vi "write_params.vi"(8 "error in (no error)":errorcluster caption="entrée d'erreur (pas d'erreur)", 10 "params":T1={"damping"=0.5, "max_iter"=200, "convergence_iter"=15, "copy"=TRUE, "preference"={"preference_type"="None", "preference_list"=[], "preference_float"=0.0}, "affinity"="euclidean", "verbose"=TRUE, "random_state"=0}, 11 "AffinityPropagation en entrée":refnum<class "AffinityPropagation.lvclass">) -> (0 "error out":errorcluster caption="sortie d'erreur", 3 "AffinityPropagation en sortie":refnum<class "AffinityPropagation.lvclass">)   [LabVIEW 2020, in "AffinityPropagation.lvclass"]
uses:
  AffinityPropagation.lvclass
  Controls/affinity_propagation_params.ctl
  AffinityPropagation.lvclass/AffinityPropagation.ctl
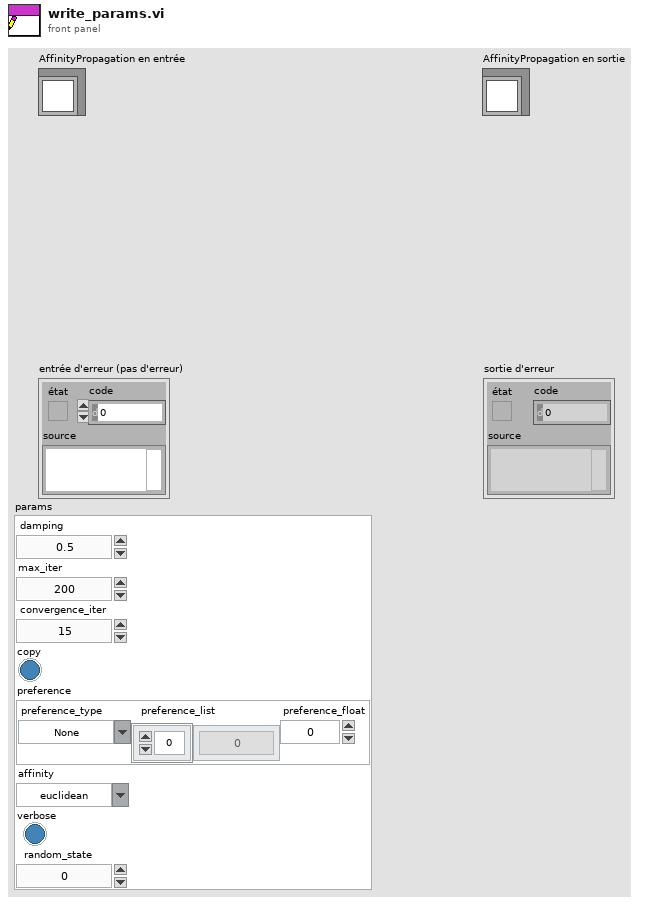
[diagram p1: front panel]
types:
  T1 = typedef "affinity_propagation_params.ctl" = cluster{"damping":dbl, "max_iter":i32, "convergence_iter":i32, "copy":bool, "preference":cluster{"preference_type":string, "preference_list":dbl[], "preference_float":dbl}, "affinity":string, "verbose":bool, "random_state":i32}
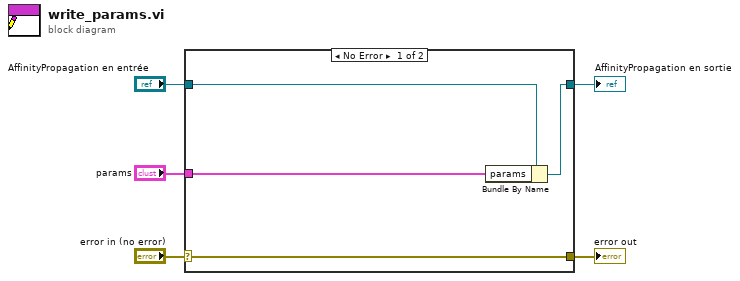
[diagram p0: block diagram]
diagram:
  n1 = case shown="No Error" "error in (no error)" {
    selector: "error in (no error)" -> [w9 w10]
    tunnel: [w9 w10] -> w4
    tunnel: [w7 w11] -> w2
    tunnel: "AffinityPropagation en entrée" -> [w8 w11]
    tunnel: "params" -> [w6 _]
    frame No Error {
      n2 = Bundle By Name(cluster=w8, "params"=w6) -> (w7:refnum<class "AffinityPropagation.lvclass">)
    }
    frame Error {
    }
  }
  "error out" <- w4
  "AffinityPropagation en sortie" <- w2
